vi "DUT Plugin MTK7615 Initialize Export.vi"(0 "Socket Parameters":cluster{"WLAN":cluster{"IP Address":string}}={"WLAN"={"IP Address"="192.168.1.1"}}, 5 "General Parameters":T3={"WLAN"={"Port Parameters Telnet"={"Bytes to Read"=1000, "Line Separator"="\n", "Port Timeout (ms)"=5000, "Read Mode"=enum."normal", "Write Mode"=enum."normal", "Remote Port"=23}, "CLI Login"={"Do Login"=TRUE, "Login Prompt"="localhost login: ", "Password"="labview", "User Name"="root"}}}, 7 "Logger":T4, 11 "error in (no error)":errorcluster) -> (4 "DUT Technology Handles":refnum<class "niDTS SystemDutHandle.lvclass">[](array[class]), 15 "Error":errorcluster)   [LabVIEW 2015, in "MTK7615.lvlib"]
uses:
  MTK7615.lvlib
  Framework/Logger/Includes/niDTS Logger INC Handle.ctl
  Framework/Logger/Objects/BASE_class/niDTS Logger.lvclass
  TestStand/Station/Objects/SystemDutHandle/niDTS SystemDutHandle.lvclass
  CommLib/Includes/niDTS Comm INC Telnet Port Parameters.ctl
  CommLib/Includes/niDTS Comm INC CLI Login.ctl
  MTK7615.lvclass
  Technologies/WLAN/Dut/Objects/BASE_class/niDTS WLAN Dut.lvclass
  CommLib/niDTS CommLib.lvlib
  Technologies/WLAN/niDTS WLAN.lvlib
  Framework/niDTS Framework.lvlib
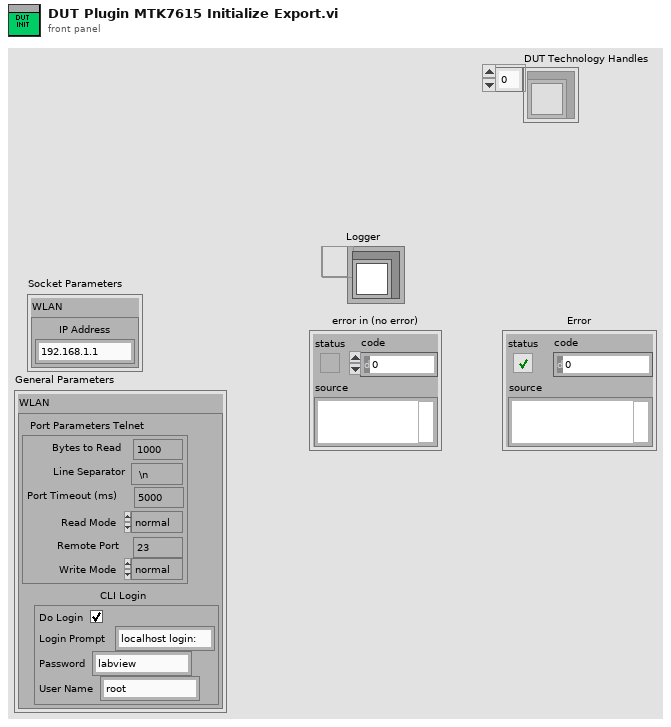
[diagram p1: front panel]
types:
  T1 = typedef "niDTS CommLib.lvlib/niDTS Comm INC Telnet Port Parameters.ctl" = cluster{"Bytes to Read":i32, "Line Separator":string, "Port Timeout (ms)":i32, "Read Mode":enum16{"normal", "line", "buffered"}, "Write Mode":enum16{"normal", "line", "buffered"}, "Remote Port":u16}
  T2 = typedef "niDTS CommLib.lvlib/niDTS Comm INC CLI Login.ctl" = cluster{"Do Login":bool, "Login Prompt":string, "Password":string, "User Name":string}
  T3 = cluster{"WLAN":cluster{"Port Parameters Telnet":T1, "CLI Login":T2}}
  T4 = typedef "niDTS Framework.lvlib/niDTS Logger INC Handle.ctl" = refnum<data-value>
  T5 = cluster{"Port Parameters Telnet":T1, "CLI Login":T2}
  T6 = typedef "niDTS CommLib.lvlib/niDTS Comm String INC Handle.ctl" = refnum<data-value>
  T7 = typedef "niDTS WLAN.lvlib/niDTS WLAN Dut INC Handle.ctl" = refnum<data-value>
  T8 = typedef "niDTS Framework.lvlib/niDTS Test INC Technology.ctl" = string
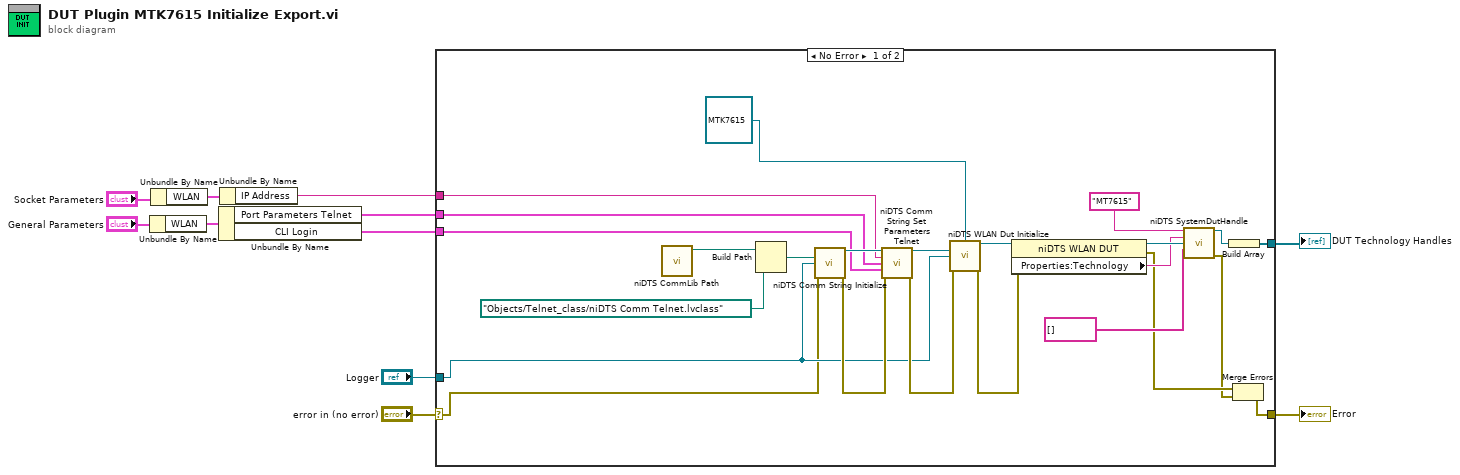
[diagram p0: block diagram]
diagram:
  n1 = Unbundle By Name("General Parameters") -> ("WLAN"=w5:T5)
  n2 = Unbundle By Name("Socket Parameters") -> ("WLAN"=w7:cluster{"IP Address":string})
  n3 = Unbundle By Name(w5) -> ("Port Parameters Telnet"=w2:T1, "CLI Login"=w1:T2)
  n4 = Unbundle By Name(w7) -> ("IP Address"=w3:string)
  n5 = case shown="No Error" "error in (no error)" {
    selector: "error in (no error)" -> [w18 w36]
    tunnel: "Logger" -> [w19 _]
    tunnel: [w17 w36] -> w10
    tunnel: [w16 _] -> w8
    tunnel: w3 -> [w15 _]
    tunnel: w2 -> [w14 _]
    tunnel: w1 -> [w13 _]
    frame No Error {
      n6 = call "niDTS CommLib Path.vi"() -> ("CommLib Path"=w20:path)  [unwired: 11 in]
      n7 = Build Path(base path=w20, name or relative path=path "Objects/Telnet_class/niDTS Comm Telnet.lvclass" ("Plugin Path")) -> (appended path=w34:path)
      n8 = call "niDTS Comm String Initialize.vi"("Plugin Path"=w34, "Logger"=w19, "error in (no error)"=w18) -> ("Comm String Handle"=w31:T6, "error out"=w29:errorcluster)  [unwired: 11 in]
      n9 = call "niDTS Comm String Set Parameters Telnet.vi"("Comm String Handle"=w31, "IP Address"=w15, "Port Parameters Telnet"=w14, "CLI Login"=w13, "error in (no error)"=w29) -> ("Comm String Handle Out"=w30:T6, "error out"=w28:errorcluster)  [unwired: 9 in]
      n10 = call "niDTS WLAN Dut Initialize.vi"("WLAN Dut Object Type"=refnum<class "MTK7615.lvclass"> refnum ("MTK7615.lvlib:MTK7615.lvclass"), "Comm Handle"=w30, "Logger"=w19, "error in (no error)"=w28) -> ("WLAN Dut Handle out"=w33:T7, "error out"=w32:errorcluster)  [unwired: 10 in]
      n11 = property class="niDTS WLAN DUT"(reference=w33, error in=w32) -> (reference out=w27:T7, error out=w23:errorcluster, "Properties:Technology"=w25:T8)
      n12 = call "niDTS SystemDutHandle.vi"("Name"="MT7615", "Technolgy"=w25, "Dut Handle"=w27, "Capabilities"=string[] []) -> ("niDTS SystemDutHandle"=w21:refnum<class "niDTS SystemDutHandle.lvclass">, "error out"=w22:errorcluster)  [unwired: 10 in]
      n13 = Build Array(w21) -> (w16:refnum<class "niDTS SystemDutHandle.lvclass">[])
      n14 = Merge Errors(w23, w22) -> (w17:errorcluster)
    }
    frame Error {
    }
  }
  "Error" <- w10
  "DUT Technology Handles" <- w8
